vi "primos.vi"(11 "Numeric":u32) -> (3 "Boolean":bool)   [LabVIEW 2015]
doc: "Este script determina si el numero indicado es un numero primo o no"
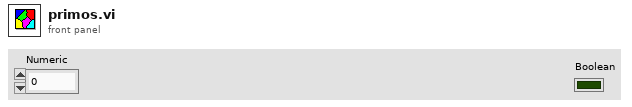
[diagram p1: front panel]
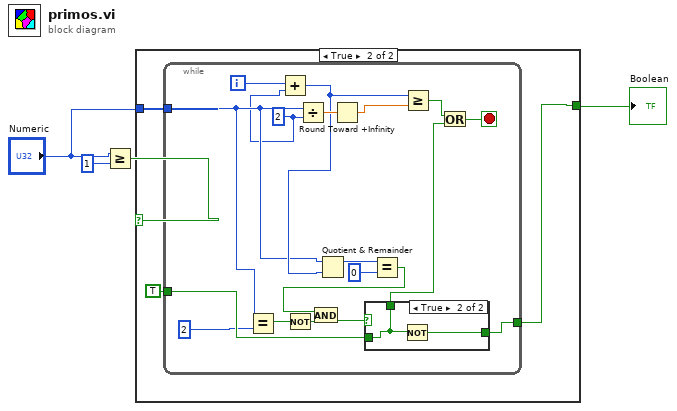
[diagram p0: block diagram]
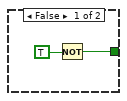
[diagram p2: hidden frame]
diagram:
  n1 = Greater Or Equal?(x="Numeric", y=u32 1) -> (x >= y?=w3:bool)
  n2 = case shown="True" w3 {
    tunnel: [w5 w7] -> w2
    tunnel: "Numeric" -> [_ w9]
    frame False {
      n3 = Not(x=TRUE) -> (.not. x?=w5:bool)
    }
    frame True {
      n4 = while {
        tunnel: w9 -> [w15]
        tunnel: TRUE -> [w24]
        tunnel: [w23] -> w7
        i -> [w16]
        stop <- w20 stop-if-true
        w11 = u32 2 ("y")
        n5 = Equal?(x=w15, y=u32 2) -> (x = y?=w12:bool)
        n6 = Add(x=w16, y=w11) -> (x+y=w19:u32)
        n7 = Not(x=w12) -> (.not. x?=w13:bool)
        n8 = Divide(x=w15, y=w11) -> (x/y=w27:dbl)
        n9 = Quotient & Remainder(x=w15, y=w19) -> (x-y*floor(x/y)=w26:u32)  [unwired: 1 out]
        n10 = Round Toward +Infinity(x=w27) -> (ceil(x): smallest int >= x=w10:dbl)
        n11 = Equal?(x=w26, y=0) -> (x = y?=w17:bool)
        n12 = And(x=w17, y=w13) -> (x .and. y?=w18:bool)
        n13 = case shown="True" w18 {
          selector: w18 -> [w28 _]
          tunnel: w24 -> [w29 w30]
          tunnel: [w29 w31] -> w23
          tunnel: [w28 w30] -> w22
          frame False {
          }
          frame True {
            n14 = Not(x=w30) -> (.not. x?=w31:bool)
          }
        }
        n15 = Greater Or Equal?(x=w19, y=w10) -> (x >= y?=w21:bool)
        n16 = Or(x=w21, y=w22) -> (x .or. y?=w20:bool)
      }
    }
  }
  "Boolean" <- w2
